vi "_get_iv_sweep3.vi"(5 "I-V class":T1={"start(mV)"=0.0, "stop(mV)"=5.0, "step(mV)"=0.1, "file_name"="IV-TRx_0.00_111_test.csv", "IF OFF/ON"=TRUE, "SAVE OFF/ON"=TRUE, "frq(GHz)"=8.0, "avg"=1, "Sweep frequency"=1, "VminfromSS"=0.05, "measurement mode"=1, "V　opt"=0} {"measurement mode" items=["Voltage sweep", "Every time HOT/COLD"]; "Sweep frequency" items=["Once", "Hot/Cold"]}, 6 "Control":T2={"GPIB_ATT"="28", "6501Dev#"=1, "GPIB_SP"="18", "GPIB_PM"="13", "GPIB_DSA"="11", "GPIB_DMM (TPD)"="23", "GPIB_MPI"="2", "motor setting"=[{"Axis"=0, "ID"=0, "HIspeed"=200.0, "LOspeed"=100.0, "ACCEL(ms)"=100.0, "Sratio"=50.0, "free run"=TRUE, "motor"="DSB HOT/COLD"}, {"Axis"=1, "ID"=0, "HIspeed"=4.0, "LOspeed"=4.0, "ACCEL(ms)"=100.0, "Sratio"=50.0, "free run"=TRUE, "motor"="SubMM Att"}], "DATA path"=path "Z:/band10/Labview_ALMA/MIX95/test", "DB path"=path "Z:/band10/Labview_ALMA/MIX95/test", "comment"="P1_Tmin", "ColdCarts"="003601", "Th"=295.0, "Tc"=77.0, "Set_SIS_volt"=2.1, "Offset"=0.0, "control"=0, "FreqLO"=800.0, "Set_Mag_Cur"=800.0, "MPI offset(mm)"=22.99, "HOT/COLD"=0} {"HOT/COLD" items=["DSB", "SBR", "GainComp"]; "control" items=["CLOSE LOOP", "OPEN LOOP", "Not Control"]}, 7 "Bias_LO_equip":T3={"Node address"=19, "CAN Interface"="CAN0", "Cartridge band"=10, "Slave Node in"={"Address"=0, "Serial Number"=[]}, "ObjHandle out"=0, "POL"=1, "sb"=1, "GPIB_SM (SIS S,V)"="24", "GPIB_DMM (SIS I)"="22", "GPIB_SM (MAG I) "="25", "GPIB_SG(LO)"="19", "GPIB_PW (PAMP) "="6", "GPIB_TMP1(8ch)"="12", "GPIB_TMP2(2ch)  "="13", "WCA_avg"=10, "Rsen"=10.0, "BiasModule"=1, "LOModule "=1, "WCA_LO_FREQ_SET"={"YTO Low freq. [GHz]"=14.42, "YTO High freq. [GHz]"=17.7, "Kvco"=1, "Lock Pol."=0, "SET LO FREQ"=72.5, "Multiplier"=6.0, "YTO (HEX)"=0, "YTO coarse( FREQ)"=25.0, "NULL PLL INTEGRATOR"=FALSE}, "Res for"=0} {"Res for" items=["none", "series res", "parallel res"]; "WCA_LO_FREQ_SET"."YTO coarse( FREQ)" min=25 max=150 step=0.0001 format="%.3f"; "WCA_LO_FREQ_SET"."Multiplier" min=3 max=6 step=3; "WCA_LO_FREQ_SET"."SET LO FREQ" min=25 max=150 step=0.0001 format="%.3f"; "WCA_LO_FREQ_SET"."Lock Pol." items=["Lower", "Upper"]; "WCA_LO_FREQ_SET"."Kvco" items=["7.5MHz/V", "15MHz/V"]; "WCA_LO_FREQ_SET"."YTO High freq. [GHz]" format="%.3f"; "WCA_LO_FREQ_SET"."YTO Low freq. [GHz]" format="%.3f"; "LOModule" items=["Manual", "B10Lab LO", "WCA LO"]; "BiasModule" items=["B10Lab Bias", "WCA BiasModule"]; "Slave Node in"."Serial Number" format="%.0x"; "Slave Node in"."Address" format="%.0x"; "Cartridge band" max=10 step=1; "Node address" format="%.0x"}) -> (1 "Vset":dbl[](array[numeric]), 2 "VP class":cluster{"array":dbl[], "array2":dbl[]}={"array"=[0.01598318, 0.06513434, 0.11293879999999999, 0.1619218, 0.2178901, 0.2672934, 0.31804370000000004, 0.367363, 0.41693539999999996, 0.4669284, 0.5198665, 0.5685969, 0.6183373000000001, 0.6677411000000001, 0.7166393999999999, 0.7705879, 0.8199078, 0.8691426999999999, 0.9186306999999999, 0.9676981, 1.017018, 1.069787, 1.119022, 1.167585, 1.217662, 1.267318, 1.319835, 1.369492, 1.4178000000000002, 1.4682140000000001, 1.517703, 1.570893, 1.6187829999999999, 1.6684379999999999, 1.718767, 1.767665, 1.817236, 1.870092, 1.919581, 1.969235, 2.017545, 2.067286, 2.120813, 2.169124, 2.220464, 2.268519, 2.318851, 2.371452, 2.4205170000000003, 2.469584, 2.5203360000000004, 2.568644, 2.618637, 2.671408, 2.72039, 2.770385, 2.819198, 2.868433, 2.9208659999999997, 2.971279, 3.0196720000000004, 3.0696679999999996, 3.118399, 3.1678, 3.22158, 3.27006, 3.319798, 3.3673480000000002, 3.4165010000000002, 3.47104, 3.5190989999999998, 3.567909, 3.617316, 3.666299, 3.718898, 3.769481, 3.8193889999999997, 3.868544, 3.9170200000000004, 3.9687819999999996, 4.019781, 4.069101000000001, 4.117915, 4.167235, 4.217732, 4.2698279999999995, 4.319991, 4.368974000000001, 4.418376, 4.4678640000000005, 4.52072, 4.569364, 4.620788, 4.669606, 4.718672, 4.768245, 4.820424999999999, 4.870415, 4.918897, 4.968636, 5.018542], "array2"=[-42.2780585, -41.3875999, -43.1175756, -42.883491, -43.0422265, -44.4769484, -43.7252964, -42.7488678, -41.2526793, -42.0770988, -42.3150146, -49.5265475, -41.4875961, -41.5542019, -44.5940842, -43.0813201, -41.8918388, -41.2766166, -44.3579354, -40.7200451, -43.9098135, -41.8305483, -43.7747917, -40.7792024, -40.9946335, -42.1528356, -41.2141044, -41.8722422, -41.8630749, -40.0888449, -41.8226515, -46.0902997, -40.6026045, -39.4622882, -41.4810266, -40.8786737, -43.7717003, -42.6439513, -42.3476097, -40.5170727, -40.3340697, -41.0877188, -42.0812836, -42.2143478, -39.9878809, -42.7571764, -42.0336087, -48.197121, -44.0607084, -42.0835869, -41.7259087, -43.0451017, -48.2958078, -42.3580828, -45.8895115, -40.6740795, -42.2677754, -41.5205874, -42.9105192, -41.5305352, -41.0601621, -40.6393958, -43.5013109, -41.8285732, -43.5176004, -41.5479038, -41.6310831, -39.9490152, -40.4863689, -50.2565085, -40.9490709, -41.8602893, -40.142096, -43.2086135, -42.3216467, -43.4879776, -47.3127246, -42.9864326, -41.7012875, -39.8670272, -42.831677, -41.940203, -41.1383045, -40.6315921, -48.2245993, -40.4902865, -42.3842672, -44.6827239, -47.9508814, -46.7971642, -42.4548707, -44.9901997, -41.1477484, -41.3566634, -41.1745101, -46.2045525, -44.6542379, -44.3579354, -40.5020576, -41.7228224, -50.7728404]}, 3 "VI class":cluster{"array":dbl[], "array2":dbl[]}={"array"=[0.01598318, 0.06513434, 0.11293879999999999, 0.1619218, 0.2178901, 0.2672934, 0.31804370000000004, 0.367363, 0.41693539999999996, 0.4669284, 0.5198665, 0.5685969, 0.6183373000000001, 0.6677411000000001, 0.7166393999999999, 0.7705879, 0.8199078, 0.8691426999999999, 0.9186306999999999, 0.9676981, 1.017018, 1.069787, 1.119022, 1.167585, 1.217662, 1.267318, 1.319835, 1.369492, 1.4178000000000002, 1.4682140000000001, 1.517703, 1.570893, 1.6187829999999999, 1.6684379999999999, 1.718767, 1.767665, 1.817236, 1.870092, 1.919581, 1.969235, 2.017545, 2.067286, 2.120813, 2.169124, 2.220464, 2.268519, 2.318851, 2.371452, 2.4205170000000003, 2.469584, 2.5203360000000004, 2.568644, 2.618637, 2.671408, 2.72039, 2.770385, 2.819198, 2.868433, 2.9208659999999997, 2.971279, 3.0196720000000004, 3.0696679999999996, 3.118399, 3.1678, 3.22158, 3.27006, 3.319798, 3.3673480000000002, 3.4165010000000002, 3.47104, 3.5190989999999998, 3.567909, 3.617316, 3.666299, 3.718898, 3.769481, 3.8193889999999997, 3.868544, 3.9170200000000004, 3.9687819999999996, 4.019781, 4.069101000000001, 4.117915, 4.167235, 4.217732, 4.2698279999999995, 4.319991, 4.368974000000001, 4.418376, 4.4678640000000005, 4.52072, 4.569364, 4.620788, 4.669606, 4.718672, 4.768245, 4.820424999999999, 4.870415, 4.918897, 4.968636, 5.018542], "array2"=[-0.0321035, -0.0223871, -0.0201793, -0.0235177, -0.019411400000000002, -0.0120628, -0.0131187, -0.018163500000000003, -0.012148099999999998, -0.013417299999999998, -0.0287331, -0.0110602, -0.014089300000000003, -0.0295651, -0.023816300000000002, -0.027687899999999998, -0.0225684, -0.0115189, -0.014633199999999999, -0.0143239, -0.017011599999999998, -0.017438299999999997, -0.030791599999999995, -0.011604199999999999, -0.0206379, -0.02003, -0.012340100000000001, -0.0215125, -0.028306500000000002, -0.0338313, -0.0283705, -0.0208939, -0.0195714, -0.0317515, -0.0174063, -0.012340100000000001, -0.0186221, -0.0212992, -0.0278372, -0.013683999999999998, -0.0108363, -0.019336700000000002, -0.0262054, -0.0105163, -0.0127134, -0.0159877, -0.0150172, -0.0159771, -0.0251388, -0.0204353, -0.0118495, -0.013758600000000001, -0.011390899999999999, -0.016553, -0.020669899999999998, -0.0207339, -0.019677999999999998, -0.013268000000000002, -0.0192194, -0.0229417, -0.029522400000000004, -0.014910499999999998, -0.009727, -0.0215339, -0.030141, -0.0086605, -0.007423300000000001, -0.0202753, -0.029511700000000002, -0.0108043, -0.0106869, -0.013833300000000001, -0.014686500000000002, -0.028957100000000003, -0.0226537, -0.01971, -0.023048400000000004, -0.0172356, -0.0249362, -0.0210006, -0.014857200000000001, -0.0273573, -0.0114442, -0.0142492, -0.0281465, -0.0081059, -0.009566999999999999, -0.034545900000000004, -0.009566999999999999, -0.0085005, -0.027378599999999996, -0.0321461, -0.0285625, 0.0047142, -0.015795800000000002, -0.031079600000000002, -0.0065593, -0.0185048, -0.015678400000000002, -0.012244099999999999, -0.023816300000000002]})   [LabVIEW 2017]
uses:
  <vilib>/express/express arith-compare/Formula/XNode/ExpressFormulaBlockNode.xnode
panel:
  out "XY graph":cluster{dbl[], dbl[]}[](graph)
  out "Measuring":u32(slide) scale=0.0..11.0
  # "LO freq. [GHz]"
  # "YTO LOW\n/High Freq."
  # "ZERO Intgrtr"
  # "Node Address"
  # "Serial Number"
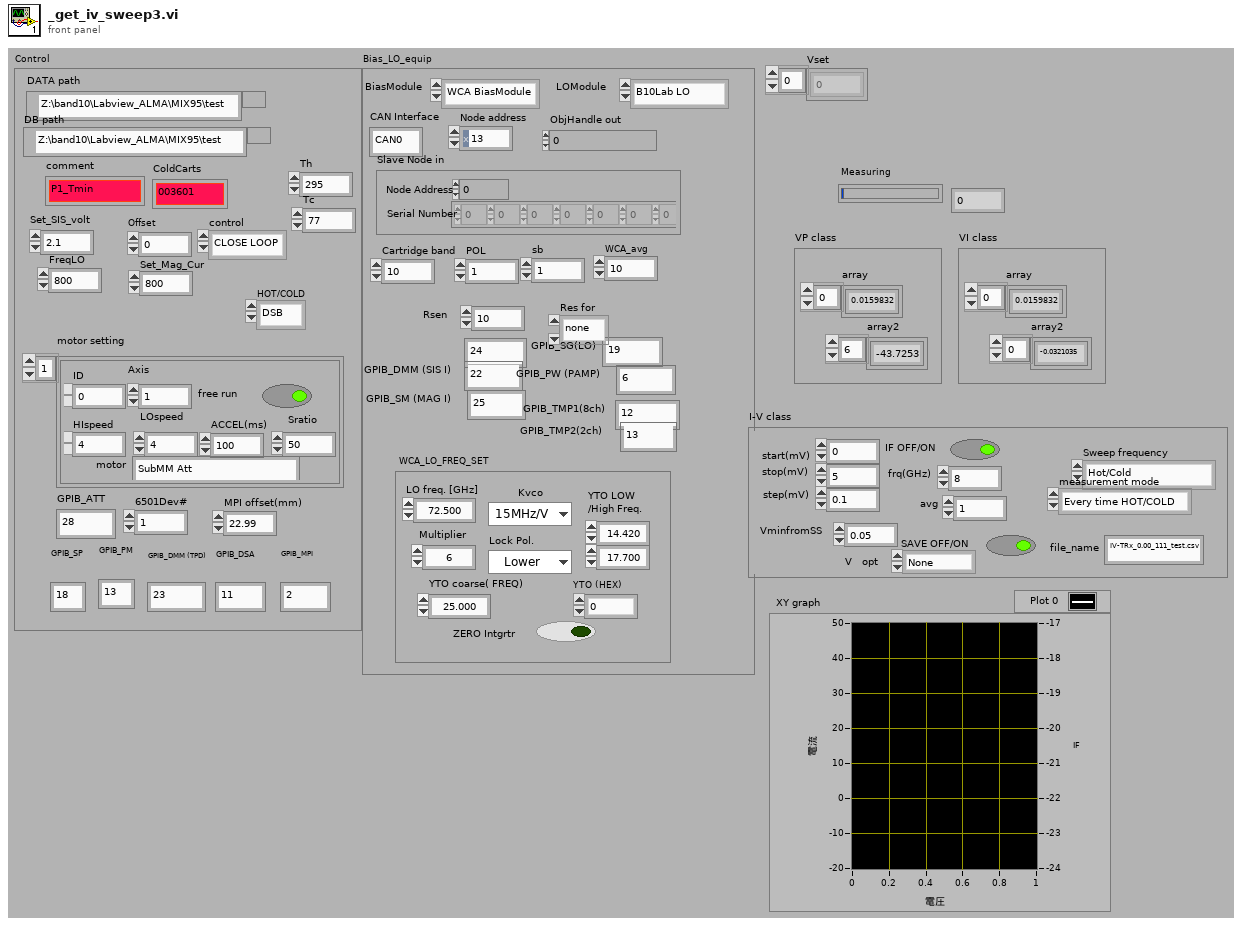
[diagram p1: front panel]
types:
  T1 = cluster{"start(mV)":dbl, "stop(mV)":dbl, "step(mV)":dbl, "file_name":string, "IF OFF/ON":bool, "SAVE OFF/ON":bool, "frq(GHz)":dbl, "avg":i32, "Sweep frequency":u16, "VminfromSS":dbl, "measurement mode":u16, "V　opt":u16}
  T2 = cluster{"GPIB_ATT":string, "6501Dev#":i16, "GPIB_SP":string, "GPIB_PM":string, "GPIB_DSA":string, "GPIB_DMM (TPD)":string, "GPIB_MPI":string, "motor setting":cluster{"Axis":i16, "ID":i16, "HIspeed":dbl, "LOspeed":dbl, "ACCEL(ms)":dbl, "Sratio":dbl, "free run":bool, "motor":string}[], "DATA path":path, "DB path":path, "comment":string, "ColdCarts":string, "Th":dbl, "Tc":dbl, "Set_SIS_volt":dbl, "Offset":dbl, "control":u16, "FreqLO":dbl, "Set_Mag_Cur":dbl, "MPI offset(mm)":dbl, "HOT/COLD":u16}
  T3 = cluster{"Node address":u16, "CAN Interface":string, "Cartridge band":u32, "Slave Node in":cluster{"Address":i16, "Serial Number":i8[]}, "ObjHandle out":u32, "POL":u32, "sb":u32, "GPIB_SM (SIS S,V)":string, "GPIB_DMM (SIS I)":string, "GPIB_SM (MAG I) ":string, "GPIB_SG(LO)":string, "GPIB_PW (PAMP) ":string, "GPIB_TMP1(8ch)":string, "GPIB_TMP2(2ch)  ":string, "WCA_avg":i32, "Rsen":dbl, "BiasModule":u16, "LOModule ":u16, "WCA_LO_FREQ_SET":cluster{"YTO Low freq. [GHz]":sgl, "YTO High freq. [GHz]":sgl, "Kvco":u16, "Lock Pol.":u16, "SET LO FREQ":sgl, "Multiplier":sgl, "YTO (HEX)":u16, "YTO coarse( FREQ)":sgl, "NULL PLL INTEGRATOR":bool}, "Res for":u16}
  T4 = cluster{"Axis":i16, "ID":i16, "HIspeed":dbl, "LOspeed":dbl, "ACCEL(ms)":dbl, "Sratio":dbl, "free run":bool, "motor":string}[]
  T5 = cluster{"Axis":i16, "ID":i16, "HIspeed":dbl, "LOspeed":dbl, "ACCEL(ms)":dbl, "Sratio":dbl, "free run":bool, "motor":string}
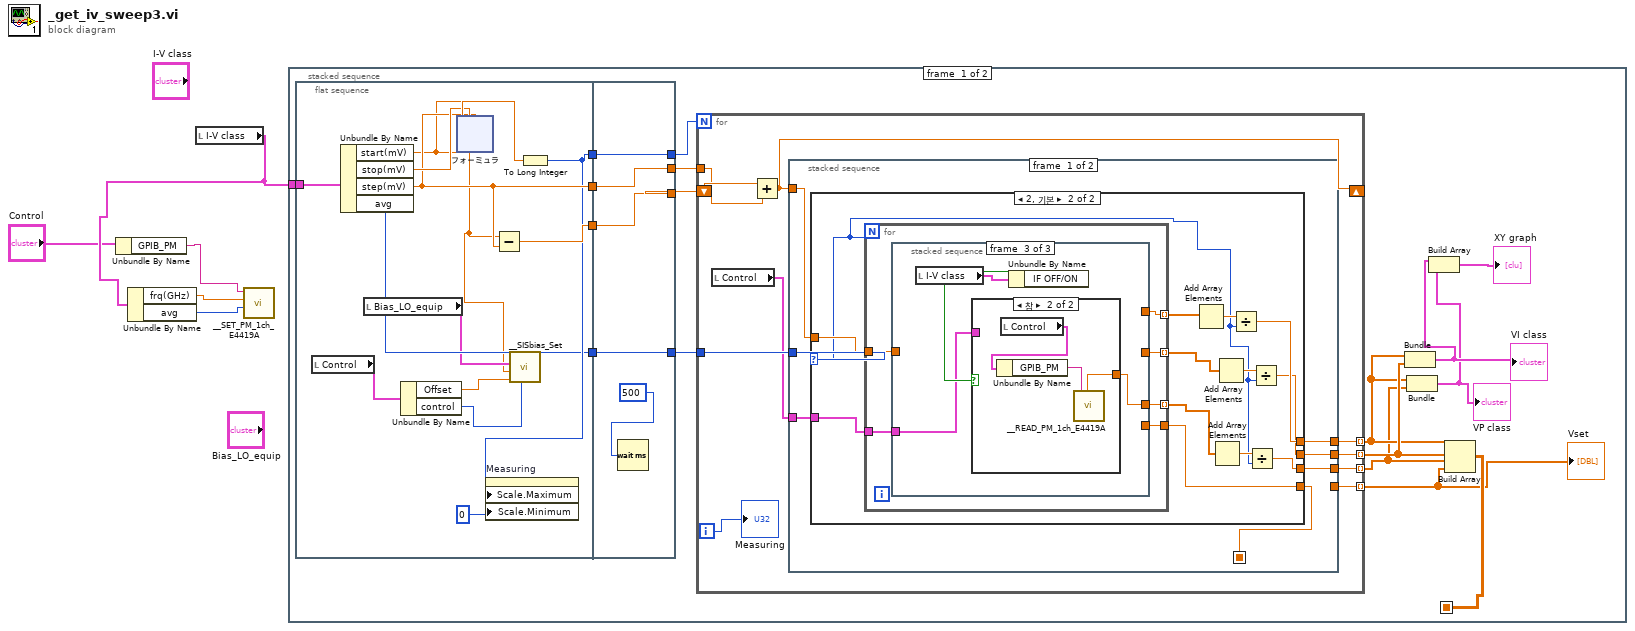
[diagram p0: block diagram]
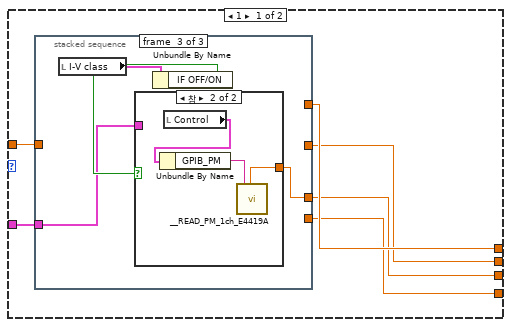
[diagram p2: hidden frame]
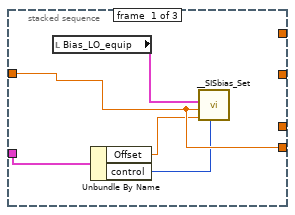
[diagram p3: hidden frame]
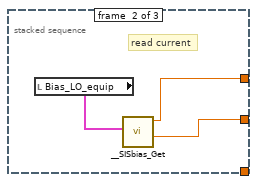
[diagram p4: hidden frame]
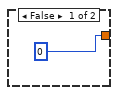
[diagram p5: hidden frame]
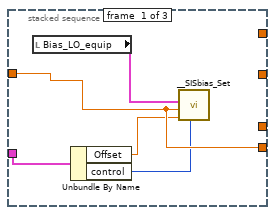
[diagram p6: hidden frame]
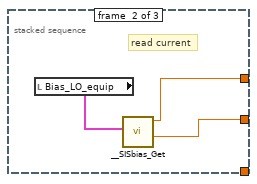
[diagram p7: hidden frame]
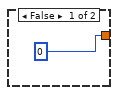
[diagram p8: hidden frame]
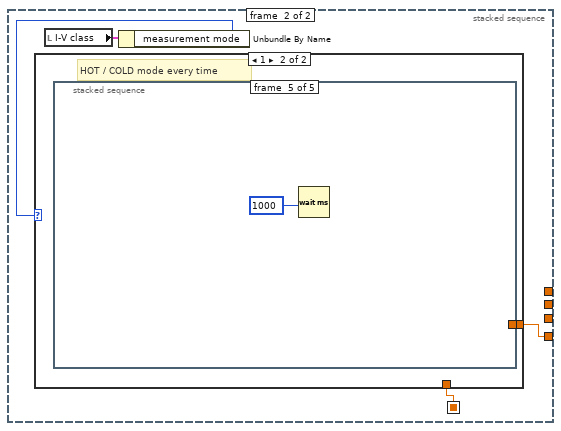
[diagram p9: hidden frame]
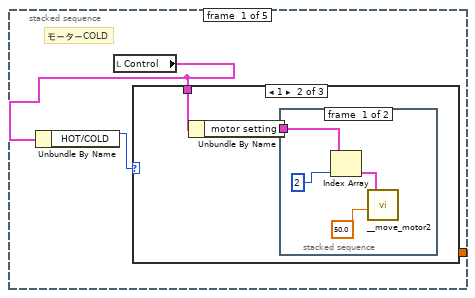
[diagram p11: hidden frame]
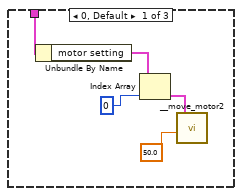
[diagram p12: hidden frame]
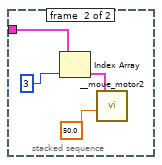
[diagram p13: hidden frame]
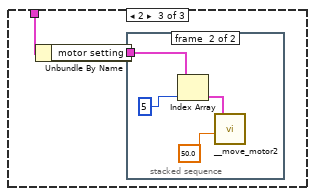
[diagram p14: hidden frame]
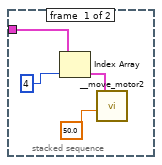
[diagram p15: hidden frame]
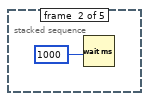
[diagram p16: hidden frame]
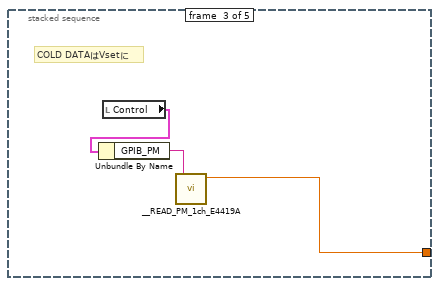
[diagram p17: hidden frame]
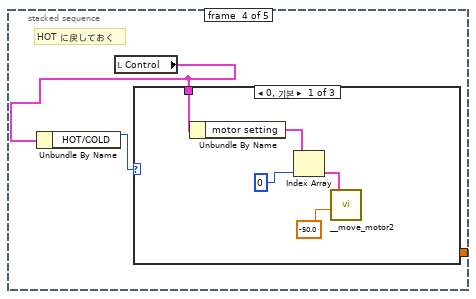
[diagram p18: hidden frame]
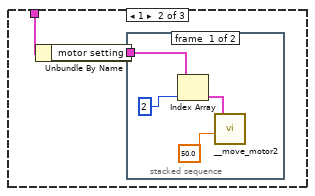
[diagram p19: hidden frame]
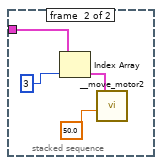
[diagram p20: hidden frame]
diagram:
  n1 = Unbundle By Name("Control") -> ("GPIB_PM"=w3:string)
  n2 = local read "I-V class"() -> (w2:T1)
  n3 = Unbundle By Name(w2) -> ("frq(GHz)"=w5:dbl, "avg"=w4:i32)
  n4 = call "__SET_PM_1ch_E4419A.VI"("aveg"=w4, "frq(GHz)"=w5, "GPIB"=w3) -> ()  [unwired: 5 in]
  n5 = stacked-sequence {
    seq-local: [w15 _] -> [_ w198]
    tunnel: w2 -> [w22 w194]
    frame #0 {
      n6 = flat-sequence {
        tunnel: w22 -> [w25]
        tunnel: [w33] -> w12
        tunnel: [w32] -> w11
        tunnel: [w31] -> w10
        tunnel: [w29] -> w9
        tunnel: [w49] -> w13
        tunnel: [w50] -> w19
        tunnel: [w51] -> w20
        tunnel: [w52] -> w21
        tunnel: w12 -> [w52]
        tunnel: w11 -> [w51]
        tunnel: w10 -> [w50]
        tunnel: w9 -> [w49]
        frame #0 {
          n7 = local read "Control"() -> (w23:T2)
          n8 = Unbundle By Name(w25) -> ("start(mV)"=w24:dbl, "stop(mV)"=w34:dbl, "step(mV)"=w32:dbl, "avg"=w29:i32)
          n9 = local read "Bias_LO_equip"() -> (w28:T3)
          n10 = Unbundle By Name(w23) -> ("Offset"=w27:dbl, "control"=w26:u16)
          n11 = xnode "フォーミュラ"("start"=w24, "stop"=w34, "step"=w32) -> ("結果"=w35:dbl)  [unwired: 1 in, 1 out]
          n12 = Subtract(x=w24, y=w32) -> (x-y=w33:dbl)
          n13 = call "__SISbias_Set.vi"("SIS　Mode"=w26, "Offset"=w27, "Set_V"=w24, "Bias_LO_equip"=w28) -> ()  [unwired: 7 in, 1 out]
          n14 = To Long Integer(number=w35) -> (32bit integer=w31:i32)
          n15 = property on="Measuring" class="Slide (决拜茄)"("Scale.Maximum"=w31, "Scale.Minimum"=0) -> ()  [unwired: 2 in, 2 out]
        }
        frame #1 {
          n16 = Wait (ms)(milliseconds to wait=500) -> ()  [unwired: 1 out]
        }
      }
      n17 = for {
        N: w19 -> [_]
        shift-right: [w60] -> _
        shift-left: w21 -> [w62]
        tunnel: w20 -> [w61]
        tunnel: [w58] -> w17 mode=indexing
        tunnel: [w57] -> w18 mode=indexing
        tunnel: [w56] -> w16 mode=indexing
        tunnel: [w55] -> w14 mode=indexing
        tunnel: w13 -> [w54]
        i -> [w59]
        n18 = local read "Control"() -> (w53:T2)
        n19 = Add(x=w62, y=w61) -> (x+y=w60:dbl)
        n20 = stacked-sequence {
          seq-local: [w63 _] -> [_ w127]
          tunnel: w60 -> [w69 _]
          tunnel: [w68 _] -> w58
          tunnel: [w67 _] -> w57
          tunnel: [w66 _] -> w56
          tunnel: [_ w128] -> w55
          tunnel: w54 -> [w65 _]
          tunnel: w53 -> [w64 _]
          frame #0 {
            n21 = case shown="2, 기본" w65 {
              selector: w65 -> [_ w93]
              tunnel: w69 -> [w75 w104]
              tunnel: w64 -> [w74 w103]
              tunnel: [w73 w99] -> w68
              tunnel: [w72 w95] -> w67
              tunnel: [w71 w94] -> w66
              tunnel: [w70 w102] -> w63
              frame 1 {
                n22 = stacked-sequence {
                  tunnel: w75 -> [w79 _ _]
                  tunnel: [_ w81 _] -> w72
                  tunnel: [_ _ w85] -> w71
                  tunnel: w74 -> [w78 _ w86]
                  tunnel: [_ w82 _] -> w73
                  tunnel: [w79 _ _] -> w70
                  frame #0 {
                    n23 = local read "Bias_LO_equip"() -> (w80:T3)
                    n24 = Unbundle By Name(w78) -> ("Offset"=w77:dbl, "control"=w76:u16)
                    n25 = call "__SISbias_Set.vi"("SIS　Mode"=w76, "Offset"=w77, "Set_V"=w79, "Bias_LO_equip"=w80) -> ()  [unwired: 7 in, 1 out]
                  }
                  frame #1 {
                    # "read current"
                    n26 = local read "Bias_LO_equip"() -> (w83:T3)
                    n27 = call "__SISbias_Get.vi"("Bias_LO_equip"=w83) -> ("Get_I(uA)"=w81:dbl, "Get_V(mV)"=w82:dbl)  [unwired: 8 in, 1 out]
                  }
                  frame #2 {
                    n28 = local read "I-V class"() -> (w84:T1)
                    n29 = Unbundle By Name(w84) -> ("IF OFF/ON"=w87:bool)
                    n30 = case shown="참" w87 {
                      tunnel: w86 -> [_ _]
                      tunnel: [0 w90] -> w85
                      frame False {
                      }
                      frame True {
                        n31 = local read "Control"() -> (w89:T2)
                        n32 = Unbundle By Name(w89) -> ("GPIB_PM"=w91:string)
                        n33 = call "__READ_PM_1ch_E4419A.VI"("GPIB"=w91) -> ("chA"=w90:dbl)  [unwired: 6 in]
                      }
                    }
                  }
                }
              }
              frame 2, Default {
                n34 = for {
                  N: w93 -> [_]
                  tunnel: w104 -> [w110]
                  tunnel: w103 -> [w109]
                  tunnel: [w108] -> w101 mode=indexing
                  tunnel: [w107] -> w96 mode=indexing
                  tunnel: [w106] -> w92 mode=indexing
                  tunnel: [w105] -> w102
                  n35 = stacked-sequence {
                    tunnel: w110 -> [w114 _ _]
                    tunnel: [_ w116 _] -> w107
                    tunnel: [_ _ w120] -> w106
                    tunnel: w109 -> [w113 _ w121]
                    tunnel: [_ w117 _] -> w108
                    tunnel: [w114 _ _] -> w105
                    frame #0 {
                      n36 = local read "Bias_LO_equip"() -> (w115:T3)
                      n37 = Unbundle By Name(w113) -> ("Offset"=w112:dbl, "control"=w111:u16)
                      n38 = call "__SISbias_Set.vi"("SIS　Mode"=w111, "Offset"=w112, "Set_V"=w114, "Bias_LO_equip"=w115) -> ()  [unwired: 7 in, 1 out]
                    }
                    frame #1 {
                      # "read current"
                      n39 = local read "Bias_LO_equip"() -> (w118:T3)
                      n40 = call "__SISbias_Get.vi"("Bias_LO_equip"=w118) -> ("Get_I(uA)"=w116:dbl, "Get_V(mV)"=w117:dbl)  [unwired: 8 in, 1 out]
                    }
                    frame #2 {
                      n41 = local read "I-V class"() -> (w119:T1)
                      n42 = Unbundle By Name(w119) -> ("IF OFF/ON"=w122:bool)
                      n43 = case shown="참" w122 {
                        tunnel: w121 -> [_ _]
                        tunnel: [0 w125] -> w120
                        frame False {
                        }
                        frame True {
                          n44 = local read "Control"() -> (w124:T2)
                          n45 = Unbundle By Name(w124) -> ("GPIB_PM"=w126:string)
                          n46 = call "__READ_PM_1ch_E4419A.VI"("GPIB"=w126) -> ("chA"=w125:dbl)  [unwired: 6 in]
                        }
                      }
                    }
                  }
                }
                n47 = Add Array Elements(numeric array=w101) -> (sum=w100:dbl)
                n48 = Add Array Elements(numeric array=w92) -> (sum=w98:dbl)
                n49 = Add Array Elements(numeric array=w96) -> (sum=w97:dbl)
                n50 = Divide(x=w100, y=w93) -> (x/y=w99:dbl)
                n51 = Divide(x=w98, y=w93) -> (x/y=w94:dbl)
                n52 = Divide(x=w97, y=w93) -> (x/y=w95:dbl)
              }
            }
          }
          frame #1 {
            n53 = local read "I-V class"() -> (w130:T1)
            n54 = Unbundle By Name(w130) -> ("measurement mode"=w129:u16)
            n55 = case shown="1" w129 {
              tunnel: [w131 w132] -> w128
              tunnel: w127 -> [w131 _]
              frame 0, Default {
                # "When the voltage is switched on\nConnect Vset as it is"
              }
              frame 1 {
                # "HOT / COLD mode every time"
                n56 = stacked-sequence {
                  tunnel: [_ _ w161 _ _] -> w132
                  frame #0 {
                    # "モーターCOLD"
                    n57 = local read "Control"() -> (w134:T2)
                    n58 = Unbundle By Name(w134) -> ("HOT/COLD"=w133:u16)
                    n59 = case shown="1" w133 {
                      tunnel: w134 -> [w137 w141 w151]
                      frame 0, Default {
                        n60 = Unbundle By Name(w137) -> ("motor setting"=w136:T4)
                        n61 = Index Array(array=w136, index=0) -> (element=w135:T5)
                        n62 = call "__move_motor2.vi"("Moving distance"=50.0, "motor setup"=w135) -> ()  [unwired: 2 in, 2 out]
                      }
                      frame 1 {
                        n63 = Unbundle By Name(w141) -> ("motor setting"=w140:T4)
                        n64 = stacked-sequence {
                          tunnel: w140 -> [w143 w147]
                          frame #0 {
                            n65 = Index Array(array=w143, index=2) -> (element=w142:T5)
                            n66 = call "__move_motor2.vi"("Moving distance"=50.0, "motor setup"=w142) -> ()  [unwired: 2 in, 2 out]
                          }
                          frame #1 {
                            n67 = Index Array(array=w147, index=3) -> (element=w146:T5)
                            n68 = call "__move_motor2.vi"("Moving distance"=50.0, "motor setup"=w146) -> ()  [unwired: 2 in, 2 out]
                          }
                        }
                      }
                      frame 2 {
                        n69 = Unbundle By Name(w151) -> ("motor setting"=w150:T4)
                        n70 = stacked-sequence {
                          tunnel: w150 -> [w154 w157]
                          frame #0 {
                            n71 = Index Array(array=w154, index=4) -> (element=w153:T5)
                            n72 = call "__move_motor2.vi"("Moving distance"=50.0, "motor setup"=w153) -> ()  [unwired: 2 in, 2 out]
                          }
                          frame #1 {
                            n73 = Index Array(array=w157, index=5) -> (element=w156:T5)
                            n74 = call "__move_motor2.vi"("Moving distance"=50.0, "motor setup"=w156) -> ()  [unwired: 2 in, 2 out]
                          }
                        }
                      }
                    }
                  }
                  frame #1 {
                    n75 = Wait (ms)(milliseconds to wait=1000) -> ()  [unwired: 1 out]
                  }
                  frame #2 {
                    # "COLD DATAはVsetに"
                    n76 = local read "Control"() -> (w162:T2)
                    n77 = Unbundle By Name(w162) -> ("GPIB_PM"=w163:string)
                    n78 = call "__READ_PM_1ch_E4419A.VI"("GPIB"=w163) -> ("chA"=w161:dbl)  [unwired: 6 in]
                  }
                  frame #3 {
                    # "HOT に戻しておく"
                    n79 = local read "Control"() -> (w165:T2)
                    n80 = Unbundle By Name(w165) -> ("HOT/COLD"=w164:u16)
                    n81 = case shown="0, 기본" w164 {
                      tunnel: w165 -> [w168 w172 w182]
                      frame 0, Default {
                        n82 = Unbundle By Name(w168) -> ("motor setting"=w167:T4)
                        n83 = Index Array(array=w167, index=0) -> (element=w166:T5)
                        n84 = call "__move_motor2.vi"("Moving distance"=-50.0, "motor setup"=w166) -> ()  [unwired: 2 in, 2 out]
                      }
                      frame 1 {
                        n85 = Unbundle By Name(w172) -> ("motor setting"=w171:T4)
                        n86 = stacked-sequence {
                          tunnel: w171 -> [w174 w178]
                          frame #0 {
                            n87 = Index Array(array=w174, index=2) -> (element=w173:T5)
                            n88 = call "__move_motor2.vi"("Moving distance"=50.0, "motor setup"=w173) -> ()  [unwired: 2 in, 2 out]
                          }
                          frame #1 {
                            n89 = Index Array(array=w178, index=3) -> (element=w177:T5)
                            n90 = call "__move_motor2.vi"("Moving distance"=50.0, "motor setup"=w177) -> ()  [unwired: 2 in, 2 out]
                          }
                        }
                      }
                      frame 2 {
                        n91 = Unbundle By Name(w182) -> ("motor setting"=w181:T4)
                        n92 = stacked-sequence {
                          tunnel: w181 -> [w185 w188]
                          frame #0 {
                            n93 = Index Array(array=w185, index=4) -> (element=w184:T5)
                            n94 = call "__move_motor2.vi"("Moving distance"=50.0, "motor setup"=w184) -> ()  [unwired: 2 in, 2 out]
                          }
                          frame #1 {
                            n95 = Index Array(array=w188, index=5) -> (element=w187:T5)
                            n96 = call "__move_motor2.vi"("Moving distance"=50.0, "motor setup"=w187) -> ()  [unwired: 2 in, 2 out]
                          }
                        }
                      }
                    }
                  }
                  frame #4 {
                    n97 = Wait (ms)(milliseconds to wait=1000) -> ()  [unwired: 1 out]
                  }
                }
              }
            }
          }
        }
        "Measuring" <- w59
      }
      "Vset" <- w14
      n98 = Bundle(w17, w18) -> (w8:cluster{dbl[], dbl[]})  [unwired: 1 in]
      "VI class" <- w8
      n99 = Bundle(w17, w16) -> (w7:cluster{dbl[], dbl[]})  [unwired: 1 in]
      "VP class" <- w7
      n100 = Build Array(w8, w7) -> (→"XY graph":cluster{dbl[], dbl[]}[])
      n101 = Build Array(w17, w18, w16, w14) -> (w15:dbl[][])
    }
    frame #1 {
      n102 = Unbundle By Name(w194) -> ("SAVE OFF/ON"=w199:bool)
      n103 = case shown="참" w199 {
        tunnel: w194 -> [_ w208]
        tunnel: w198 -> [_ w206]
        tunnel: w194 -> [_ _]
        frame False {
        }
        frame True {
          n104 = local read "Control"() -> (w200:T2)
          n105 = Unbundle By Name(w200) -> ("Offset"=w202:dbl)
          n106 = Unbundle By Name(w208) -> ("file_name"=w207:string)
          n107 = Format Into String(format string="V(mV),I(uA),P(dBm),Vset with Offset=%f", w202) -> (resulting string=w204:string)  [unwired: 2 in, 1 out]
          n108 = Unbundle By Name(w200) -> ("DATA path"=w201:path)
          n109 = call "___save_2d_data_with_header.vi"("ヘッダー"=w204, "配列"=w206, "形式"="%^.3e", "file_name"=w207, "パス"=w201) -> ()  [unwired: 6 in, 1 out]
        }
      }
      n110 = local read "Control"() -> (w192:T2)
      n111 = local read "Bias_LO_equip"() -> (w197:T3)
      n112 = Unbundle By Name(w192) -> ("Set_SIS_volt"=w193:dbl, "Offset"=w196:dbl, "control"=w195:u16)
      n113 = call "__SISbias_Set.vi"("SIS　Mode"=w195, "Offset"=w196, "Set_V"=w193, "Bias_LO_equip"=w197) -> ()  [unwired: 7 in, 1 out]
    }
  }
